vi "Log Model State.vi"(8 "error in":errorcluster, 10 "Message Data":variant) -> (0 "error out":errorcluster)   [LabVIEW 2015, in "Logger.lvlib"]
uses:
  Logger.lvlib
  support/Message Queue/Message Queue.lvlib
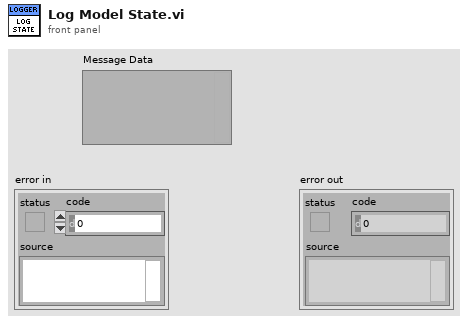
[diagram p1: front panel]
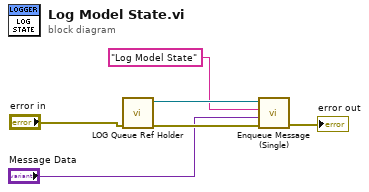
[diagram p0: block diagram]
diagram:
  n1 = call "LOG Queue Ref Holder.vi"("error in"="error in") -> ("error out"=w5:errorcluster, "Input Message Queue"=w6:refnum<queue>)  [unwired: 9 in]
  n2 = call "Enqueue Message (Single).vi"("error in (no error)"=w5, "Message Data"="Message Data", "Message"="Log Model State", "Message Queue"=w6) -> ("error out"=→"error out":errorcluster)  [unwired: 6 in, 1 out]
